vi "Write Paths Settings.vi"(8 "error in (no error)":errorcluster, 10 "PathsUpdated":T1, 11 "Tool Data in":refnum<class "Tool Data.lvclass">) -> (0 "error out":errorcluster, 3 "Tool Data out":refnum<class "Tool Data.lvclass">)   [LabVIEW 2019, in "Tool Data.lvclass"]
uses:
  Tool Data.lvclass
  Settings/Setting Database/Typedefs/PublicEvents--Setting Database.PathsUpdated.ctl
  Settings/Path Settings/Path Settings.lvclass
  Tool Data.lvclass/Tool Data.ctl
  Settings/Setting Database/Setting Database.lvclass
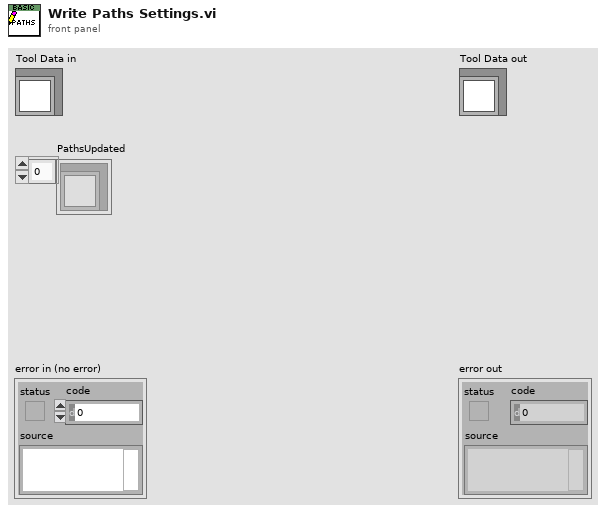
[diagram p1: front panel]
types:
  T1 = typedef "Setting Database.lvclass/PublicEvents--Setting Database.PathsUpdated.ctl" = refnum<class "Path Settings.lvclass">[]
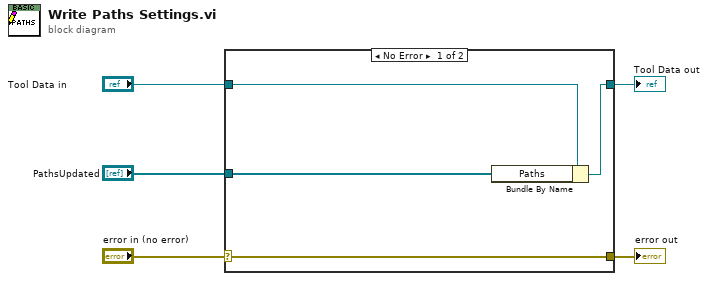
[diagram p0: block diagram]
diagram:
  n1 = case shown="No Error" "error in (no error)" {
    selector: "error in (no error)" -> [w9 w10]
    tunnel: [w9 w10] -> w4
    tunnel: [w7 w11] -> w2
    tunnel: "Tool Data in" -> [w8 w11]
    tunnel: "PathsUpdated" -> [w6 _]
    frame No Error {
      n2 = Bundle By Name(cluster=w8, "Paths"=w6) -> (w7:refnum<class "Tool Data.lvclass">)
    }
    frame Error {
    }
  }
  "error out" <- w4
  "Tool Data out" <- w2
